vi "hse-application_VersionNumber--constant.vi"() -> (3 "HSE-Libraries Version Number":string="unreleased")   [LabVIEW 2020, in "hse-application.lvclass"]
doc: "____\nHAMPEL SOFTWARE ENGINEERING v3.8.0 (2023-12-18 14:41)"
uses:
  hse-application.lvclass
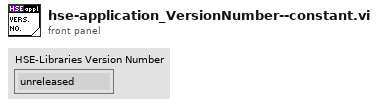
[diagram p1: front panel]
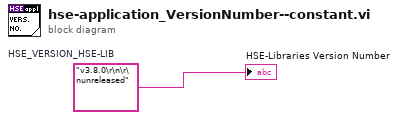
[diagram p0: block diagram]
diagram:
  w1 = "v3.8.0\r\n\r\nunreleased"  # HSE_VERSION_HSE-LIB
  "HSE-Libraries Version Number" <- w1
